vi "Init XNET Commands Session.vi"(8 "error in (no error)":errorcluster, 11 "DUT Sample in":refnum<class "DUT Sample.lvclass">) -> (0 "error out":errorcluster, 3 "DUT Sample out":refnum<class "DUT Sample.lvclass">)   [LabVIEW 2023, in "DUT Sample.lvclass"]
uses:
  DUT Sample.lvclass
  DUT Sample.lvclass/DUT Sample.ctl
  <resource>/objmgr/xnet.rc
  <vilib>/xnet/xnet.llb/XNET Create Session (Signal Input Single-point).vi
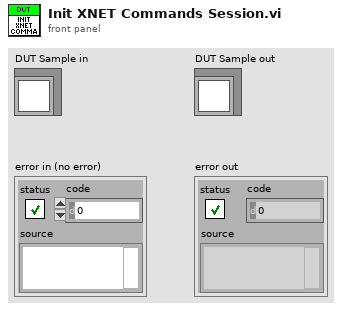
[diagram p1: front panel]
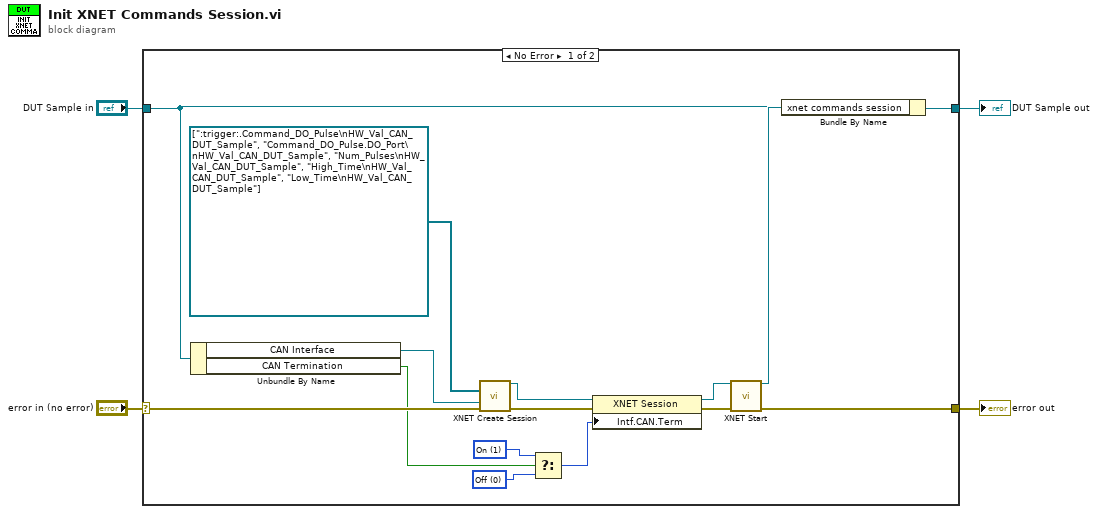
[diagram p0: block diagram]
diagram:
  n1 = case shown="No Error" "error in (no error)" {
    selector: "error in (no error)" -> [w18 w21]
    tunnel: [w17 w21] -> w3
    tunnel: [w16 w20] -> w1
    tunnel: "DUT Sample in" -> [w14 w20]
    frame No Error {
      w7 = u32 1 items=["Off", "On"] ("Interface:CAN:Termination")
      w9 = u32 0 items=["Off", "On"] ("Interface:CAN:Termination")
      n2 = Unbundle By Name(w14) -> ("CAN Interface"=w13:refnum<k21>, "CAN Termination"=w8:bool)
      n3 = call-poly <vilib>:"XNET Create Session.vi"("signal list"=refnum<k21>[] [":trigger:.Command_DO_Pulse\nHW_Val_CAN_DUT_Sample", "Command_DO_Pulse.DO_Port\nHW_Val_CAN_DUT_Sample", "Num_Pulses\nHW_Val_CAN_DUT_Sample", "High_Time\nHW_Val_CAN_DUT_Sample", "Low_Time\nHW_Val_CAN_DUT_Sample"] ("Select Signal List from database"), "interface"=w13, "error in (no error)"=w18) -> ("session out"=w11:refnum<k21>, "error out"=w19:errorcluster)  [unwired: 11 out]
      n4 = Select(t=w7, s=w8, f=w9) -> (s? t:f=w6:u32)
      n5 = property class="XNET Session"(reference=w11, error in=w19, "Intf.CAN.Term"=w6) -> (reference out=w10:refnum<k21>, error out=w12:errorcluster)
      n6 = call <vilib>:"XNET Start.vi"("session in"=w10, "error in (no error)"=w12) -> ("session out"=w15:refnum<k21>, "error out"=w17:errorcluster)  [unwired: 12 in]
      n7 = Bundle By Name(cluster=w14, "xnet commands session"=w15) -> (w16:refnum<class "DUT Sample.lvclass">)
    }
    frame Error {
    }
  }
  "error out" <- w3
  "DUT Sample out" <- w1
